vi "Global_Var_Drive.vi"() -> ()   [LabVIEW 2016]
panel:
  out "Comp_Robot?":bool
  out "Joysick2_Unassigned":bool
  out "Joystick_GearChute":bool
  out "Joystick_Feed_F":bool
  out "Joysitick_Feed_B":bool
  out "Joystick_Intake_B":bool
  out "Joystick_GateClamp":bool
  out "Joystick_GateClose":bool
  out "Joystick_GateOpen":bool
  out "Joystick_BotFeed_B":bool
  out "Joystick_BotFeed_F":bool
  in  "Joystick2_Unassigned":dbl
  in  "Joystick_Climb_UpDown":dbl
  in  "Joystick_Turret_L/R":dbl
  in  "Joystick_GearRail_R/L":dbl
  out "Joysick_Lightshow":bool
  out "Joystick_Aim":bool
  out "Joysick_Shoot":bool
  out "Joystick_Shift":bool
  out "Joystick_Unassigned":bool
  out "Joystick_Place_Gear":bool
  out "Joystick_DriveStraight":bool
  out "Joystick_Climb":bool
  out "Extra_Motor_3":bool
  out "Extra_Motor_2":bool
  out "Extra_Motor_1":bool
  out "Joystick_Gearpusher":bool
  out "Joystick_Intake":bool
  in  "Joysick_Unassigned":dbl
  in  "Joystick_F/B":dbl
  in  "Joystick_L/R_Turn":dbl
  in  "Joystick_Unassigned":dbl
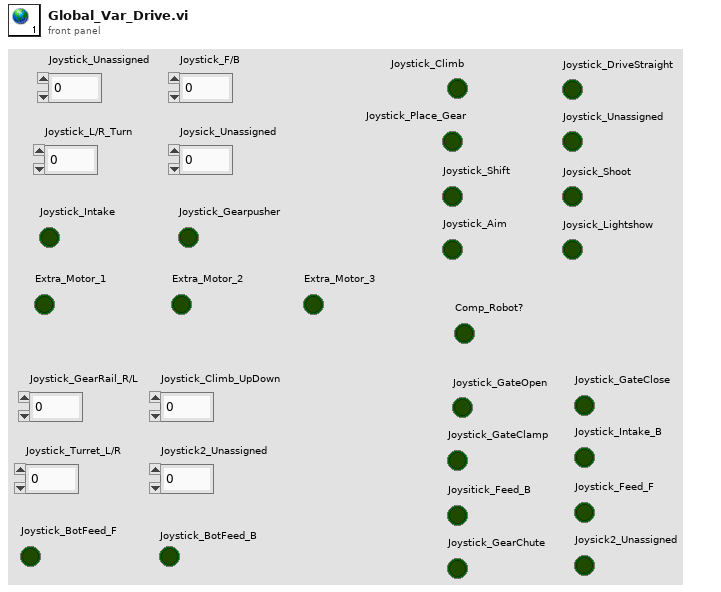
[diagram p1: front panel]
diagram:
